vi "GEA2_CMD_UPDATE_MODE.vi"(0 "ComPort":refnum<visa-resource-name>="COM3", 5 "Mode":T1=enum."HighDemand", 7 "V.Days":u8=180, 9 "V.Temp":u8=100, 11 "Error In":errorcluster) -> (4 "ACK":bool, 6 "CRC Match":bool, 15 "Error Out":errorcluster)   [LabVIEW 2014]
uses:
  Utility/GEA2 Commands/HEWH/Type Definitions/GEA2 Commands HEWH Mode.ctl
  Utility/GEA2 Commands/HEWH/Type Definitions/GEA2 Commands HEWH Command Type.ctl
panel:
  out "DataReturned":u8[](array[numeric]) format="%.0x"
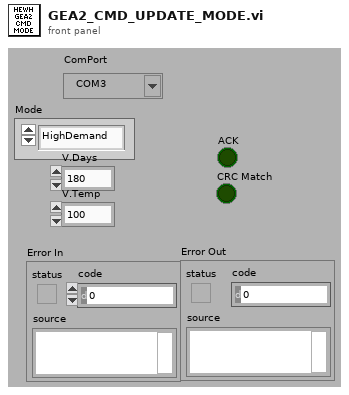
[diagram p1: front panel]
types:
  T1 = typedef "GEA2 Commands HEWH Mode.ctl" = enum16{"Hybrid", "Std Electric", "eHeat", "HighDemand", "Vacation"}
  T2 = typedef "GEA2 Commands HEWH Command Type.ctl" = u8
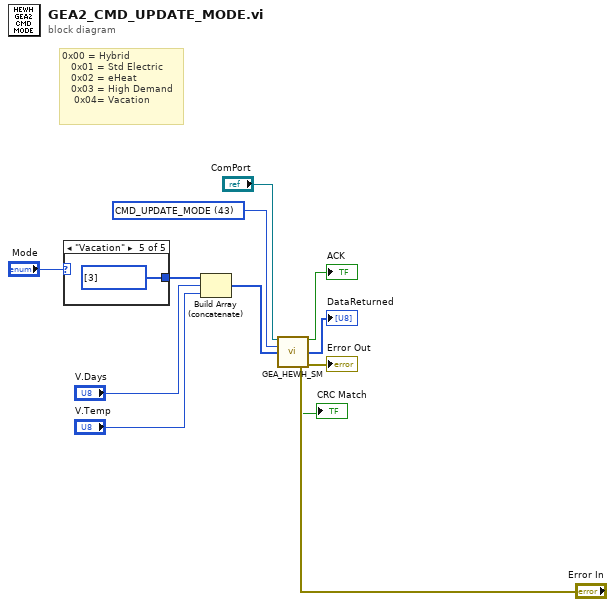
[diagram p0: block diagram]
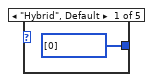
[diagram p2: hidden frame]
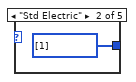
[diagram p3: hidden frame]
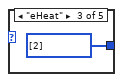
[diagram p4: hidden frame]
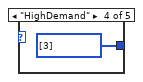
[diagram p5: hidden frame]
diagram:
  w1 = T2 43 items=["RQST_SOFTWARE_VERSION", "RQST_T2_RESISTANCE", "RQST_T3A_RESISTANCE", "RQST_T3B_RESISTANCE", "RQST_T4_RESISTANCE", "RQST_T5_RESISTANCE", "RQST_IDLB_RESISTANCE", "RQST_MODE_SELECT_RESISTANCE", "RQST_DATA_FROM_MEMORY", "RQST_DATA_FROM_DATA_FLASH", "RQST_SS_FAULT_COUNTS", "RQST_OTHER_FAULT_COUNTS", "CMD_CLEAR_FAULT_COUNTS", "RQST_HYPERTERM_OUTPUT_DATA", "CMD_RESET_FILTER_TIMES", "CMD_WRITE_SETPOINTS", "CMD_TURN_ON_OFF_DLB", "CMD_ENTER_EXIT_FCT_MODE", "CMD_SET_LEDS", "CMD_SET_EEV_DRIVE_LINES", "REQ_READ_KEY_STATUS", "RQST_READ_PERSONALITY", "CMD_ENTER_FACT_MODE", "CMD_RESET", "CMD_RESTORE_EEPROM_DEFAULTS", "CMD_SET_MODEL_NUMBER", "CMD_SET_SERIAL_NUMBER", "RQST_MODEL_NUMBER", "RQST_SERIAL_NUMBER", "CMD_TOGGLE_SERVICE_MODE", "CMD_TOGGLE_UE_SERV", "CMD_TOGGLE_LE_SERV", "CMD_REFRESH_SERVICE_TIMEOUTS", "RQST_DSM_OVERRIDE_STATUS", "RQST_STATUS_QUERY", "RQST_HEM_KWH_DATA", "RQST_SERVICE_ERROR_CODES", "RQST_OVERRIDE_STATUS", "CMD_UPDATE_DSM_LEVEL", "CMD_OVERRIDE_STATUS_CHANGED", "CMD_CLEAR_OVERRIDE_STATUS", "CMD_CLEAR_ENERGY_USAGE_CTRS", "CMD_DSM_OVERRIDES", "CMD_UPDATE_MODE", "CMD_SET_PID_P_DENOMINATOR", "CMD_SET_PID_I_DENOM_UNDER_THR", "CMD_SET_PID_I_DENOM_OVER_THR", "CMD_SET_START_POS_UNDER_THR", "CMD_SET_START_POS_OVER_THR", "CMD_SET_EEV_STOP_POSITION", "CMD_SET_AMBIENT_THRESH_1", "CMD_SET_AMBIENT_THRESH_2", "CMD_SET_AMBIENT_THRESH_3", "CMD_SET_PID_LOW_SH_TARGET", "CMD_SET_PID_MID_SH_TARGET", "RQST_PID_PARAMETERS", "CMD_COMP_OFF", "CMD_TOGGLE_FAN", "CMD_RQST_LED_STATUS", "CMD_UE_2_SECONDS", "CMD_LE_2_SECONDS", "CMD_COMP_ON", "CMD_HP_RUN_6MIN", "RQST_TEMP_RANGE", "RQST_VACATION_RANGE", "RQST_STD_ELEC_RANGE", "RQST_WATER_CAPACITY", "CMD_CANCEL_EEV_POSITION", "CMD_EEV_POSITION", "CMD_SET_CURRENTS", "RQST_SUPPORTED_MODES"] ("Command")
  # "0x00 = Hybrid\n   0x01 = Std Electric\n   0x02 = eHeat\n   0x03 = High Demand\n    0x04= Vacation"
  n1 = case shown="\"Vacation\"" "Mode" {
    tunnel: [u8[] [0] ("Command Data") u8[] [1] ("Command Data") u8[] [2] ("Command Data") u8[] [3] ("Command Data") u8[] [3] ("Command Data")] -> w7
    frame "Hybrid", Default {
    }
    frame "Std Electric" {
    }
    frame "eHeat" {
    }
    frame "HighDemand" {
    }
    frame "Vacation" {
    }
  }
  n2 = Build Array (concatenate)(w7, "V.Days", "V.Temp") -> (w4:u8[])
  n3 = call "GEA_HEWH_SM.vi"("ComPort"="ComPort", "Command"=w1, "Command Data"=w4, "Error In"="Error In") -> ("WriteACK"=→"ACK":bool, "DataReturned"=→"DataReturned":u8[], "CRC Match"=→"CRC Match":bool, "Error Out"=→"Error Out":errorcluster)  [unwired: 7 in, 1 out]
